vi "moveToPosition.vi"(0 "Controller in":refnum<class "_Controller.lvclass">, 2 "target(s) (in)":T1[](array[typedef]), 5 "error in (no error)":errorcluster) -> (14 "Controller out":refnum<class "_Controller.lvclass">, 17 "success?":bool, 18 "response":string, 19 "error out":errorcluster)   [LabVIEW 2013, in "classes.lvlib" / "_Controller.lvclass"]
doc: "Instructs the controller to move to all target values of each specified axis. The input \"target(s)\" is an array of target components. Populate that array with the appropriate axes and target position for those axes.\n\nFor example, if it's desirable to move axes X and Z to targets 256 and 10245 respectively, the input array would consist of two values:\n\nindex[0] --> [axis:X, target:256]\nindex[1] --> [axis:Z, target:10245]\n\nIf the referenced controller happens to be a single axis controller, then there only needs to be one element in the array with a specified target. Note, in this case, the actual axis is ignore; target is all that's of interest.\n\nNOTE: This VI serves as an abstract method to the Controller class. This means it exists for the sole purpose of being overridden by its sub classes (a requirement of the object oriented model).\n\nProduced By:\n\n<B>Kod Integrations, LLC</B>\n4835 Marianne Drive\nMount Airy, MD 21771\nhttp://www.kodintegrations.com\nemail: info@kodintegrations.com\nphone: (240) 687-1288"
uses:
  _Controller.lvclass
  common/controls/movement_item.ctl
  common/controls/axis.ctl
  libraries/common.lvlib
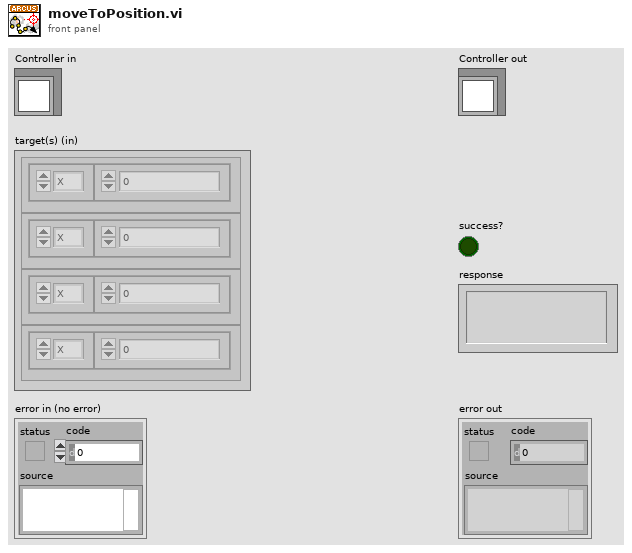
[diagram p1: front panel]
types:
  T1 = typedef "common.lvlib/movement_item.ctl" = cluster{"axis":T2, "target":i32}
  T2 = typedef "common.lvlib/axis.ctl" = enum16{"X", "Y", "Z", "U"}
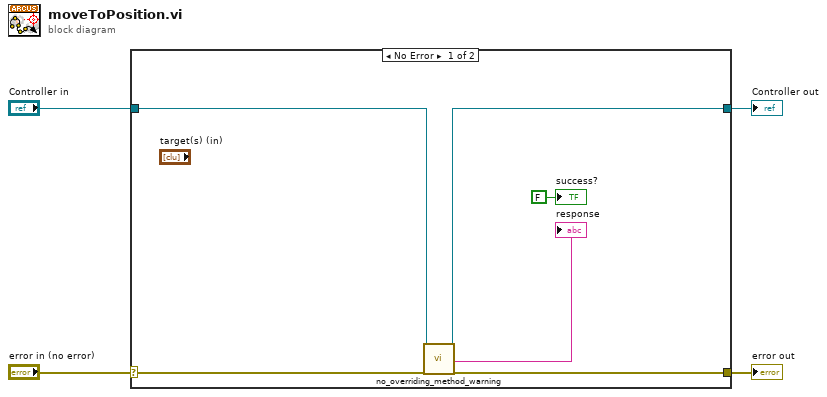
[diagram p0: block diagram]
diagram:
  n1 = case shown="No Error" "error in (no error)" {
    selector: "error in (no error)" -> [w10 w12]
    tunnel: [w9 w12] -> w3
    tunnel: [w7 w11] -> w1
    tunnel: "Controller in" -> [w8 w11]
    frame No Error {
      n2 = call "no_overriding_method_warning.vi"("Controller (in)"=w8, "error in (no error)"=w10) -> ("Controller (out)"=w7:refnum<class "_Controller.lvclass">, "msg"=→"response":string, "error out"=w9:errorcluster)  [unwired: 15 in]
      "success?" <- FALSE ("success?")
    }
    frame Error {
    }
  }
  "error out" <- w3
  "Controller out" <- w1
